vi "Property Node (Session).vi"   [LabVIEW 2020, in "NI_SFTP.lvlib"]
doc: "Gets (reads) or sets (writes) properties of an SFTP Session object. Use these properties to configure SFTP before and during a connection to an SFTP server."
uses:
  <vilib>/net/SFTP/NI_SFTP.lvlib
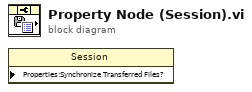
[diagram p0: block diagram]
diagram:
  n1 = property class="Session" props=["Properties:Synchronize Transferred Files?"]() -> ()  [unwired: 3 in, 2 out]
